vi "DmgrGetDvc.vi"(8 "Error In":errorcluster, 10 "Device Number":i32, 11 "Device Handle":u64) -> (0 "Error Out":errorcluster, 1 "Connection String":string, 2 "Name":string, 3 "Device Handle":u64, 4 "DTP":u32)   [LabVIEW 2011, in "LVH-Adept.lvlib" / "DMGR.lvlib"]
doc: "Get Device Handle"
uses:
  DMGR.lvlib
  Private/Type Defs/Error.ctl
  <vilib>/Utility/importsl/GetValueByPointer/datatype.ctl
  <vilib>/Utility/importsl/GetValueByPointer/GetValueByPointer.xnode
  Resources/dmgr.dll
  Program Files (x86)/National Instruments/LabVIEW 2011/resource/lvimptsl.dll
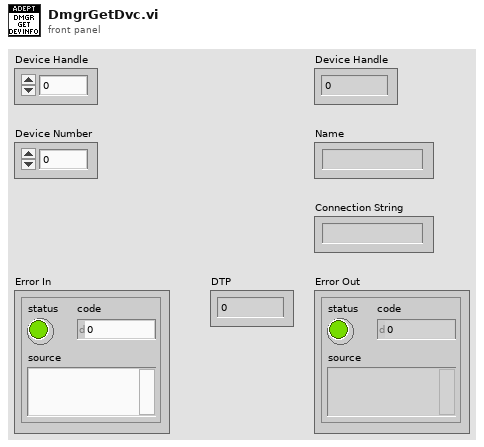
[diagram p1: front panel]
types:
  T1 = typedef "LVH-Adept.lvlib/DMGR.lvlib/Error.ctl" = enum16{"Unknown Error", "Device Enumeration", "Device Handle", "Device Info", "Device Open"}
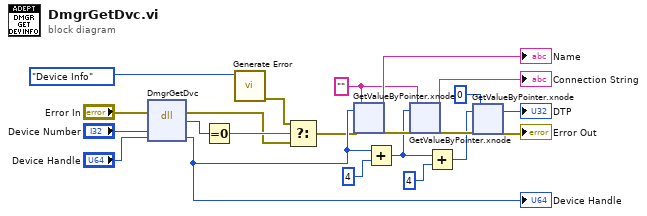
[diagram p0: block diagram]
diagram:
  w5 = ""
  n1 = dll-call lib="C:/github/labviewhacker/LVH-Adept/LabVIEW/vi.lib/LabVIEW Hacker/Adept/Private/Resources/dmgr.dll" fn="DmgrGetDvc"(error in="Error In", "Device Number"="Device Number", "deviceHandlePtr"="Device Handle") -> (error out=w17:errorcluster, "Success"=w21:u8, "deviceHandlePtr"=w4:u64)  [unwired: 3 in, 1 out]
  "Device Handle" <- w4
  n2 = Equal To 0?(x=w21) -> (x = 0?=w20:bool)
  n3 = call "Generate Error.vi"("Error Type"=Error."Device Info") -> ("Error Out"=w18:errorcluster)  [unwired: 10 in]
  n4 = Select(t=w18, s=w20, f=w17) -> (s? t:f=w2:errorcluster)
  n5 = xnode "GetValueByPointer.xnode"("Pointer"=w4, "InputType"=w5, "ErrorIn"=w2) -> ("Output"=→"Name":string, "ErrorOut"=w13:errorcluster)  [unwired: 1 in]
  n6 = Add(x=w4, y=u64 4) -> (x+y=w9:u64)
  n7 = xnode "GetValueByPointer.xnode"("Pointer"=w9, "InputType"=w5, "ErrorIn"=w13) -> ("Output"=→"Connection String":string, "ErrorOut"=w12:errorcluster)  [unwired: 1 in]
  n8 = Add(x=w9, y=u64 4) -> (x+y=w8:u64)
  n9 = xnode "GetValueByPointer.xnode"("Pointer"=w8, "InputType"=u32 0 ("y"), "ErrorIn"=w12) -> ("Output"=→"DTP":u32, "ErrorOut"=→"Error Out":errorcluster)  [unwired: 1 in]
